vi "Aufschaltung_Popup.vi"() -> ()   [LabVIEW 2020, in "CalGas Aufschaltung.lvlib"]
uses:
  CalGas Aufschaltung.lvlib
  Aufschaltung CalGas_ANZEIGE.ctl
  Visualisierungs Elemente/Auswahlfeld.ctl
  FGV CalGas Aktionen.ctl
  Sprachverwaltung/FGV Aktion Tabelle zerlegen.ctl
  Funktionstasten/Funktionstasten-Aktion.ctl
  Funktionstasten/Zustaende.ctl
  PNS/Aktionen FGV Grenzwerte.ctl
  Sprachverwaltung/Sprachverwaltung.lvlib
  Funktionstasten/Funktionstasten.lvlib
  PNS/PNS.lvlib
  Allgemein/allgemeine Sub-VIs.lvlib
panel:
  in  "Aufschaltung CalGas":T1 {"Analysator" items=["FT-IR"]; "Aufschaltpunkt" items=["Filterblock", "Analysator direkt", "PNS", "Entnahme"]; "Kalibriergas" items=["Nitrogen", "Span 1", "Span 2", "Span 3", "Span 4", "Span 5", "Span 6", "Span 7", "Span 8"]}
  # "Aufschaltung Kalibriergas"
  # "Kalibriergas"
  # "Aufschaltpunkt"
  # "Analysator"
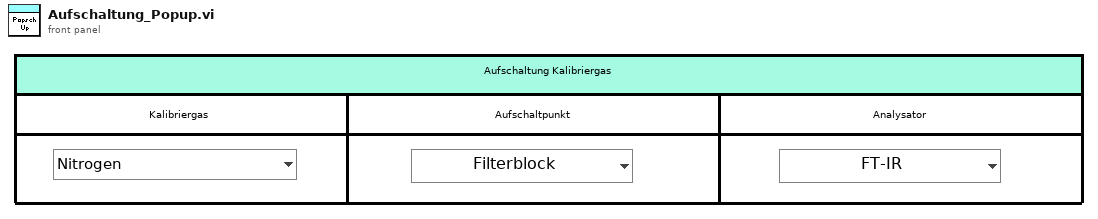
[diagram p1: front panel]
types:
  T1 = typedef "CalGas Aufschaltung.lvlib/Aufschaltung CalGas_ANZEIGE.ctl" = cluster{"Kalibriergas":T2, "Aufschaltpunkt":T2, "Analysator":T2}
  T2 = typedef "Auswahlfeld.ctl" = u16
  T3 = typedef "CalGas Aufschaltung.lvlib/FGV CalGas Aktionen.ctl" = enum16{"lesen", "Analysator Auswahl", "Def.CalGas", "Aufschaltung CalGas", "laden", "speichern", "KAL extrahieren"}
  T4 = typedef "Sprachverwaltung.lvlib/FGV Aktion Tabelle zerlegen.ctl" = enum16{"laden", "vereinzeln", "speichern"}
  T5 = enum32{"Invalid", "Default", "Floating", "Floating/Auto-Hide", "Modal"}
  T6 = typedef "CalGas Aufschaltung.lvlib/Aufschaltung CalGas.ctl" = cluster{"Kalibriergas":T2, "Aufschaltpunkt":T7, "Analysator":T8}
  T7 = typedef "CalGas Aufschaltung.lvlib/Auswahl Aufschaltpunkt.ctl" = enum16{"über Filterblock", "Analysator direkt", "über PNS", "Entnahme", "Gasdivider"}
  T8 = typedef "CalGas Aufschaltung.lvlib/Auswahl Analysator.ctl" = enum16{"FT-IR", "FID", "PMA", "PMA/FID/FT-IR"}
  T9 = typedef "CalGas Aufschaltung.lvlib/Definition CalGas Anzeige.ctl" = cluster{"Namen":T10, "Werte":T12, "Werte 2":T12, "Einheit":T14, "Messbereiche":T15}
  T10 = typedef "CalGas Aufschaltung.lvlib/CalGas-Namen.ctl" = cluster{"Name":T11, "Name 2":T11, "Name 3":T11, "Name 4":T11, "Name 5":T11, "Name 6":T11, "Name 7":T11, "Name 8":T11, "Name 9":T11, "Name 10":T11, "Name 11":T11, "Name 12":T11}
  T11 = typedef "String - Eingabefeld.ctl" = string
  T12 = typedef "CalGas Aufschaltung.lvlib/CalGas-Werte.ctl" = cluster{"Konzentration 1":T13, "Konzentration 2":T13, "Konzentration 3":T13, "Konzentration 4":T13, "Konzentration 5":T13, "Konzentration 6":T13, "Konzentration 7":T13, "Konzentration 8":T13, "Konzentration 9":T13, "Konzentration 10":T13, "Konzentration 11":T13, "Konzentration 12":T13}
  T13 = typedef "Zahlen-Eingabefeld.ctl" = sgl
  T14 = typedef "CalGas Aufschaltung.lvlib/CalGas-Einheit.ctl" = cluster{"Einheit 1":T2, "Einheit 2":T2, "Einheit 3":T2, "Einheit 4":T2, "Einheit 5":T2, "Einheit 6":T2, "Einheit 7":T2, "Einheit 8":T2, "Einheit 9":T2, "Einheit 10":T2, "Einheit 11":T2, "Einheit 12":T2}
  T15 = typedef "CalGas Aufschaltung.lvlib/CalGas-Messbereiche.ctl" = cluster{"Messbereich 1":T2, "Messbereich 2":T2, "Messbereich 3":T2, "Messbereich 4":T2, "Messbereich 5":T2, "Messbereich 6":T2, "Messbereich 7":T2, "Messbereich 8":T2, "Messbereich 9":T2, "Messbereich 10":T2, "Messbereich 11":T2, "Messbereich 12":T2}
  T16 = typedef "LVRectTypeDef.ctl" = cluster{"Left":i16, "Top":i16, "Right":i16, "Bottom":i16}
  T17 = typedef "Funktionstasten.lvlib/Zustaende.ctl" = enum16{"Standby", "Pause", "Eco", "Messen", "Kalibrieren", "Spülen Filter", "Spülen Leitung", "Umgebungsluft", "0-Gas", "Cal-Gas", "CG zu PNS", "-------------", "Init 1", "Init 2", "Init 3", "Init 4", "Messen vorbereiten", "Messen durchführen", "Exit"}
  T18 = typedef "Funktionstasten.lvlib/Funktionstasten-Aktion.ctl" = enum16{"Initialisieren", "Zustand setzen", "Taste gedrückt", "Fehler speichern", "Lesen", "Manuell", "Remote", "Bitparallel", "Samplepoint", "Zeit Prüfen", "reset Umschalten"}
  T19 = typedef "PNS.lvlib/Aktionen FGV Grenzwerte.ctl" = enum16{"lesen", "Grenzw. schreiben", "Anweisungscode", "IP-Adresse", "laden", "speichern", "Anweisungscode vorgeben"}
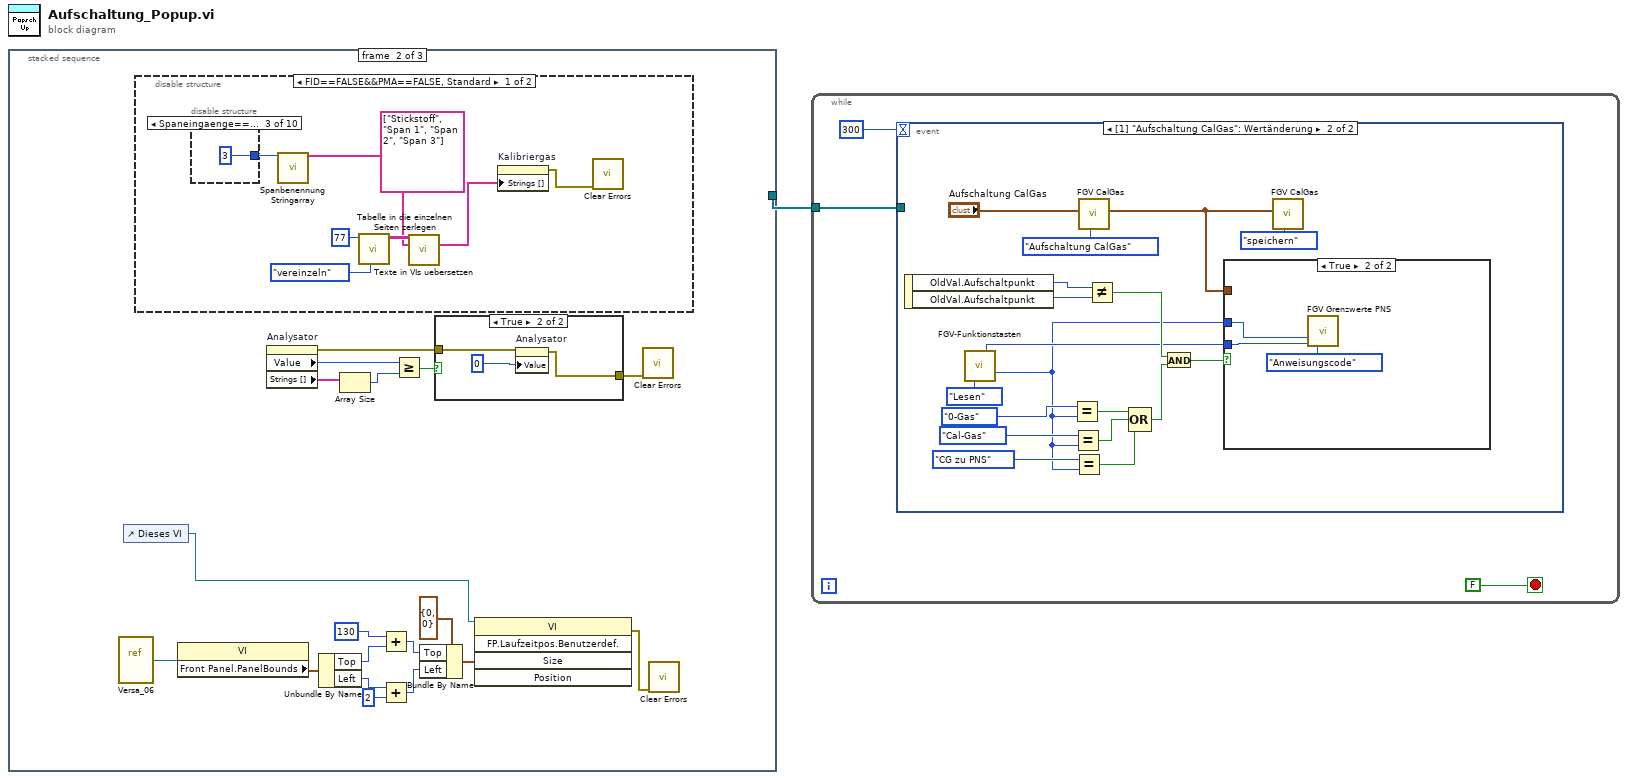
[diagram p0: block diagram]
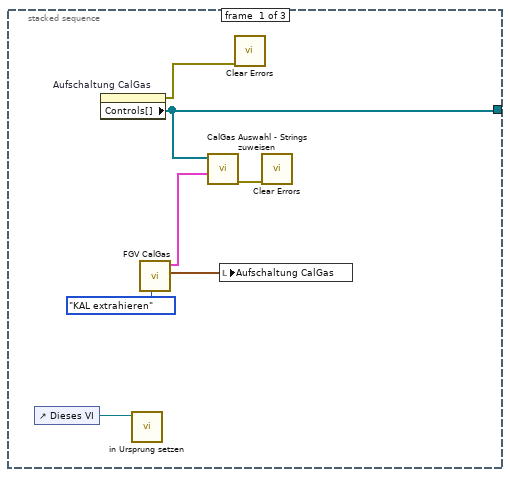
[diagram p2: hidden frame]
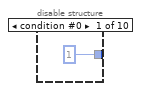
[diagram p4: hidden frame]
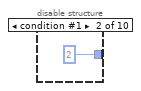
[diagram p5: hidden frame]
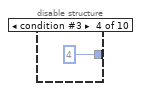
[diagram p6: hidden frame]
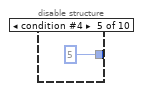
[diagram p7: hidden frame]
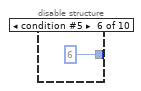
[diagram p8: hidden frame]
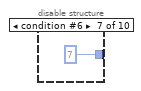
[diagram p9: hidden frame]
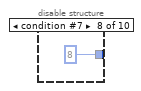
[diagram p10: hidden frame]
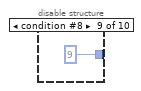
[diagram p11: hidden frame]
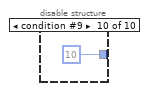
[diagram p12: hidden frame]
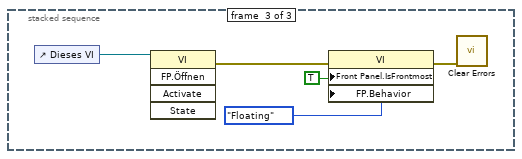
[diagram p14: hidden frame]
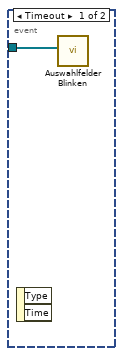
[diagram p15: hidden frame]
diagram:
  n1 = stacked-sequence {
    tunnel: [w7 _ _] -> w1
    frame #0 {
      n2 = control-ref of="Dieses VI"() -> (w2:refnum<vi>)
      n3 = property on="Aufschaltung CalGas" class="Cluster (strikt)"() -> (error out=w8:errorcluster, "Controls[]"=w7:refnum<vi>[])  [unwired: 2 in, 1 out]
      n4 = call "in Ursprung setzen.vi"("VI Referenz"=w2) -> ()  [unwired: 10 in, 1 out]
      n5 = call "FGV CalGas.vi"("Aktionen"=FGV_CalGas_Aktionen."KAL extrahieren") -> ("Aufschaltung CalGas"=w4:T6, "Def.CalGas"=w3:T9)  [unwired: 6 in, 3 out]
      n6 = call "CalGas Auswahl - Strings zuweisen.vi"("Def.CalGas"=w3, "Aufschaltung CalGas"=w7) -> ("Fehler (Ausgang)"=w6:errorcluster)  [unwired: 9 in]
      n7 = local write "Aufschaltung CalGas"(w4) -> ()
      n8 = call <vilib>:"Clear Errors.vi"("error in (no error)"=w8) -> ()  [unwired: 5 in, 2 out]
      n9 = call <vilib>:"Clear Errors.vi"("error in (no error)"=w6) -> ()  [unwired: 5 in, 2 out]
    }
    frame #1 {
      n10 = vi-ref "Versa_06.vi"() -> (w19:refnum<vi>)
      n11 = control-ref of="Dieses VI"() -> (w20:refnum<vi>)
      n12 = disable-structure shown="FID==FALSE&&PMA==FALSE, Standard" {
        frame condition #0 (active) {
          (unwired) string[] ["Stickstoff", "Span 1", "Span 2", "Span 3"] ("Strings []")
          n13 = disable-structure shown="Spaneingaenge==3" {
            disable-tunnel: [1 ("Spangaseingänge") 2 ("Spangaseingänge") 3 ("Spangaseingänge") 4 ("Spangaseingänge") 5 ("Spangaseingänge") 6 ("Spangaseingänge") 7 ("Spangaseingänge") 8 ("Spangaseingänge") 9 ("Spangaseingänge") 10 ("Spangaseingänge")] -> w31
            frame condition #0 {
            }
            frame condition #1 {
            }
            frame condition #2 (active) {
            }
            frame condition #3 {
            }
            frame condition #4 {
            }
            frame condition #5 {
            }
            frame condition #6 {
            }
            frame condition #7 {
            }
            frame condition #8 {
            }
            frame condition #9 {
            }
          }
          n14 = call "Spanbenennung Stringarray.vi"("Spangaseingänge"=w31) -> ("Span Eingänge"=w32:string[])  [unwired: 13 in, 1 out]
          n15 = call "Tabelle in die einzelnen Seiten zerlegen.vi"("Aktion"=FGV_Aktion_Tabelle_zerlegen."vereinzeln", "Index (Seite)"=77) -> ("Sprachliste"=w34:string[][])  [unwired: 7 in, 2 out]
          n16 = call "Texte in VIs uebersetzen.vi"("Sprachliste"=w34, "String-Array zum Übersetzen"=w32) -> ("String-Array zum Übersetzen"=w33:string[])  [unwired: 9 in, 4 out]
          n17 = property on="Kalibriergas" class="Ring (strikt)"("Strings []"=w33) -> (error out=w37:errorcluster)  [unwired: 2 in, 1 out]
          n18 = call <vilib>:"Clear Errors.vi"("error in (no error)"=w37) -> ()  [unwired: 5 in, 2 out]
        }
        frame condition #1 {
        }
      }
      n19 = property class="VI"(reference=w19) -> ("Front Panel.PanelBounds"=w18:T16)  [unwired: 1 in, 2 out]
      n20 = property on="Analysator" class="Ring (strikt)"() -> (error out=w22:errorcluster, "Value"=w25:T2, "Strings []"=w26:string[])  [unwired: 2 in, 1 out]
      n21 = Unbundle By Name(w18) -> ("Top"=w17:i16, "Left"=w16:i16)
      n22 = Array Size(array=w26) -> (size(s)=w24:i32)
      n23 = Add(x=i16 130, y=w17) -> (x+y=w14:i16)
      n24 = Add(x=w16, y=i16 2) -> (x+y=w12:i16)
      n25 = Greater Or Equal?(x=w25, y=w24) -> (x >= y?=w23:bool)
      n26 = Bundle By Name(cluster=cluster{"Top":i16, "Left":i16} {"Top"=0, "Left"=0} ("Position"), "Top"=w14, "Left"=w12) -> (w11:cluster{"Top":i16, "Left":i16})
      n27 = case shown="True" w23 {
        tunnel: w22 -> [w27 w29]
        tunnel: [w27 w28] -> w21
        frame False {
        }
        frame True {
          n28 = property on="Analysator" class="Ring (strikt)"(error in=w29, "Value"=0) -> (error out=w28:errorcluster)  [unwired: 1 in, 1 out]
        }
      }
      n29 = invoke class="VI" method="FP.Laufzeitpos.Benutzerdef."(reference=w20, "Size"=w11) -> (error out=w10:errorcluster)  [unwired: 3 in, 4 out]
      n30 = call <vilib>:"Clear Errors.vi"("error in (no error)"=w21) -> ()  [unwired: 5 in, 2 out]
      n31 = call <vilib>:"Clear Errors.vi"("error in (no error)"=w10) -> ()  [unwired: 5 in, 2 out]
    }
    frame #2 {
      n32 = control-ref of="Dieses VI"() -> (w48:refnum<vi>)
      n33 = invoke class="VI" method="FP.Öffnen"(reference=w48) -> (error out=w49:errorcluster)  [unwired: 4 in, 4 out]
      n34 = property class="VI"(error in=w49, "Front Panel.IsFrontmost"=TRUE ("Frontpanel-Fenster:Ist im Vordergrund"), "FP.Behavior"=T5."Floating" ("Frontpanel-Fenster:Verhaltensweise")) -> (error out=w51:errorcluster)  [unwired: 1 in, 1 out]
      n35 = call <vilib>:"Clear Errors.vi"("error in (no error)"=w51) -> ()  [unwired: 5 in, 2 out]
    }
  }
  n36 = while {
    tunnel: w1 -> [w53]
    stop <- FALSE stop-if-true
    n37 = event shown="[1] \"Aufschaltung CalGas\": Wertänderung" {
      selector: _ -> [_ _]
      dyn-events: _ -> [_ _]
      timeout: 300 -> [_ _]
      tunnel: w53 -> [w56 _]
      event Timeout {
        n38 = event-data() -> ()  [unwired: 1 in, 2 out]
        n39 = call "Auswahlfelder Blinken.vi"("Controls[]"=w56) -> ()  [unwired: 11 in]
      }
      event Value Change {
        n40 = event-data() -> ("OldVal.Aufschaltpunkt"=w72:T2, "OldVal.Aufschaltpunkt"=w60:T2)  [unwired: 1 in]
        n41 = call "FGV-Funktionstasten.vi"("Aktion"=Funktionstasten-Aktion."Lesen") -> ("Samplepoint"=w61:u16, "ausgewählte Funktion"=w59:T17)  [unwired: 7 in, 6 out]
        n42 = Equal?(x=Zustaende."0-Gas" ("y"), y=w59) -> (x = y?=w67:bool)
        n43 = Equal?(x=Zustaende."Cal-Gas" ("y"), y=w59) -> (x = y?=w66:bool)
        n44 = Equal?(x=Zustaende."CG zu PNS" ("y"), y=w59) -> (x = y?=w65:bool)
        n45 = call "FGV CalGas.vi"("Aktionen"=FGV_CalGas_Aktionen."Aufschaltung CalGas", "Aufschaltung CalGas"="Aufschaltung CalGas") -> ("Aufschaltung CalGas"=w57:T6)  [unwired: 5 in, 4 out]
        n46 = Not Equal?(x=w72, y=w60) -> (x != y?=w64:bool)
        n47 = Compound Arithmetic op=OR ("Mehrfacharithmetik")(w67, w66, w65) -> (w63:bool)
        n48 = And(x=w64, y=w63) -> (x .and. y?=w62:bool)
        n49 = case shown="True" w62 {
          tunnel: w61 -> [_ w76]
          tunnel: w59 -> [_ w75]
          tunnel: w57 -> [_ _]
          frame False {
          }
          frame True {
            n50 = call "FGV Grenzwerte PNS.vi"("Zustand"=w75, "Samplepoint"=w76, "Aktionen FGV Grenzwerte"=Aktionen_FGV_Grenzwerte."Anweisungscode") -> ()  [unwired: 10 in, 3 out]
          }
        }
        n51 = call "FGV CalGas.vi"("Aktionen"=FGV_CalGas_Aktionen."speichern", "Aufschaltung CalGas"=w57) -> ()  [unwired: 5 in, 5 out]
      }
    }
  }
